vi "TDMStoAVIGUI.vi"(0 "TDMS Path":path, 1 "Codec":string, 5 "AVI Out Path":path, 7 "Frames Per Second":u32, 11 "error in (no error)":errorcluster, 12 "Quality":i32, 13 "Image Type":u16) -> (15 "error out":errorcluster)   [LabVIEW 2023]
uses:
  Program Files/NI/LVAddons/niimaqdx/1/examples/Vision Acquisition/NI-IMAQdx/Stream to Disk/SubVIs/TDMS File Initialization (Read).vi
panel:
  in  "Stop Conversion":bool
  out "Percent Done":dbl
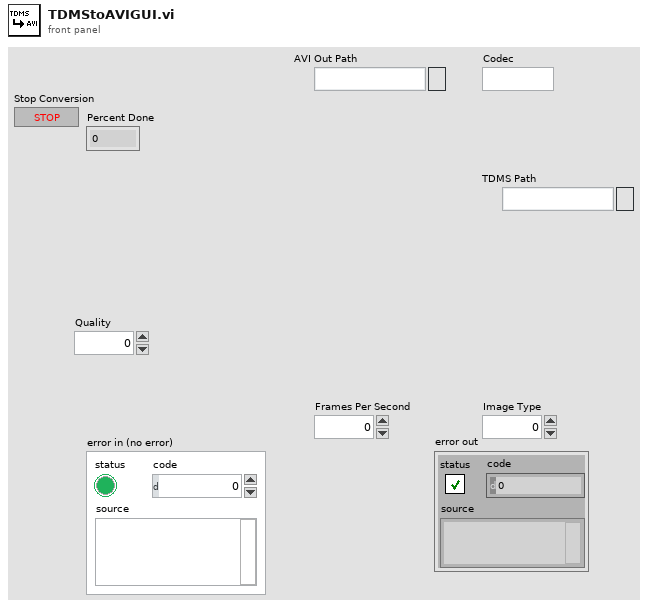
[diagram p1: front panel]
types:
  T1 = typedef "IMAQ Image.ctl" = refnum<image>
  T2 = typedef "TDMS Read Data.ctl" = cluster{"Image Type":T3, "Width":u32, "Height":u32, "Pixels per Image":u32, "Total Width":u32, "Left Offset":u32, "Image":T1}
  T3 = typedef "Image Type" = u32
  T4 = typedef "IMAQ AVI2 Refnum.ctl" = refnum<k20>
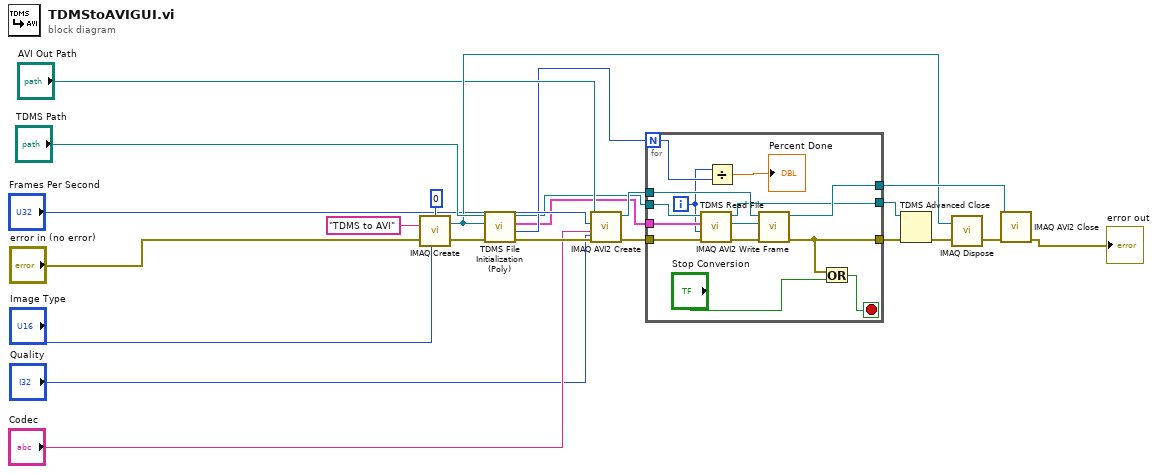
[diagram p0: block diagram]
diagram:
  n1 = call "IMAQ Create"("Border Size"=0, "Image Name"="TDMS to AVI", "Image Type"="Image Type", "error in (no error)"="error in (no error)") -> ("New Image"=w19:T1, "error out"=w13:errorcluster)  [unwired: 1 out]
  n2 = call-poly "TDMS File Initialization (Poly).vi"("error in (no error)"=w13, "Image In"=w19, "File Path"="TDMS Path") -> ("error out"=w23:errorcluster, "Number of Images in TDMS File"=w5:u32, "Read Settings"=w4:T2, "TDMS Refnum Out"=w3:refnum<k34>)  [unwired: 5 in]
  n3 = call "IMAQ AVI2 Create"("Quality"="Quality", "error in (no error)"=w23, "Codec"="Codec", "Frames Per Second"="Frames Per Second", "AVI Path"="AVI Out Path") -> ("error out"=w9:errorcluster, "AVI Refnum"=w8:T4)  [unwired: 5 in]
  n4 = for {
    N: w5 -> [w31]
    tunnel: w9 -> [w37]
    tunnel: w3 -> [w36]
    tunnel: w4 -> [w35]
    tunnel: w8 -> [w34]
    tunnel: [w26] -> w15
    tunnel: [w32] -> w20
    tunnel: [w29] -> w16
    i -> [w27]
    stop <- w24 stop-if-true
    n5 = call "TDMS Read File.vi"("error in"=w37, "Image Index"=w27, "Read Settings"=w35, "TDMS Refnum In"=w36) -> ("error out"=w33:errorcluster, "Image"=w28:T1, "TDMS Refnum Out"=w29:refnum<k34>)  [unwired: 4 in, 1 out]
    n6 = Divide(x=w27, y=w31) -> (x/y=→"Percent Done":dbl)
    n7 = call "IMAQ AVI2 Write Frame"("error in (no error)"=w33, "Image"=w28, "AVI Refnum"=w34) -> ("error out"=w26:errorcluster, "AVI Refnum (duplicate)"=w32:T4)  [unwired: 6 in, 1 out]
    n8 = Or(x=w26, y="Stop Conversion") -> (x .or. y?=w24:bool)
  }
  n9 = TDMS Advanced Close(8:w15, 11:w16) -> (0:w17:errorcluster)  [unwired: 2 in, 1 out]
  n10 = call "IMAQ Dispose"("Image"=w19, "error in (no error)"=w17) -> ("error out"=w18:errorcluster)  [unwired: 4 in]
  n11 = call "IMAQ AVI2 Close"("error in (no error)"=w18, "AVI Refnum"=w20) -> ("error out"=→"error out":errorcluster)  [unwired: 9 in]
